vi "AddNewBins.vi"(8 "error in (no error)":errorcluster, 11 "Node Ptr":u64 format="%.0x") -> (0 "error out":errorcluster)   [LabVIEW 2012, in "Histogram Custom Device.lvlib"]
uses:
  Histogram Custom Device.lvlib
  <vilib>/NI Veristand/Custom Device API/Custom Device API.lvlib
  <vilib>/NI Veristand/Custom Device API/Custom Device Channel Type.ctl
  <vilib>/NI Veristand/Custom Device API/Custom Device Channel.ctl
  BinBounds.ctl
  <vilib>/NI Veristand/Custom Device API/Set Item Property (Variant).vi
panel:
  in  "Tag":string
  # "We cant add bins individually,\nwe have to delete all of the existing \nbins and then create new ones"
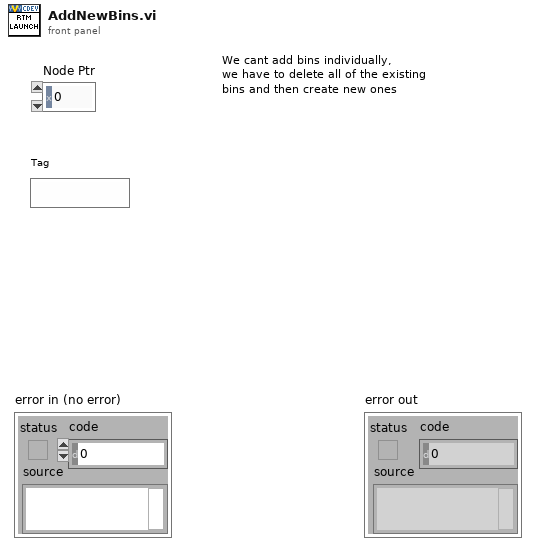
[diagram p1: front panel]
types:
  T1 = typedef "Custom Device API.lvlib/Custom Device Channel.ctl" = cluster{"Type":T2, "Units":string, "Default Value":dbl, "Faultable":bool, "Scalable":bool}
  T2 = typedef "Custom Device API.lvlib/Custom Device Channel Type.ctl" = enum16{"Input", "Output"}
  T3 = typedef "Histogram Custom Device.lvlib/BinBounds.ctl" = cluster{"Bin Counts":i32[], "Upper Bounds":dbl[], "Lower Bounds":dbl[]}
  T4 = typedef "Custom Device API.lvlib/Custom Device Item Ref.ctl" = u64
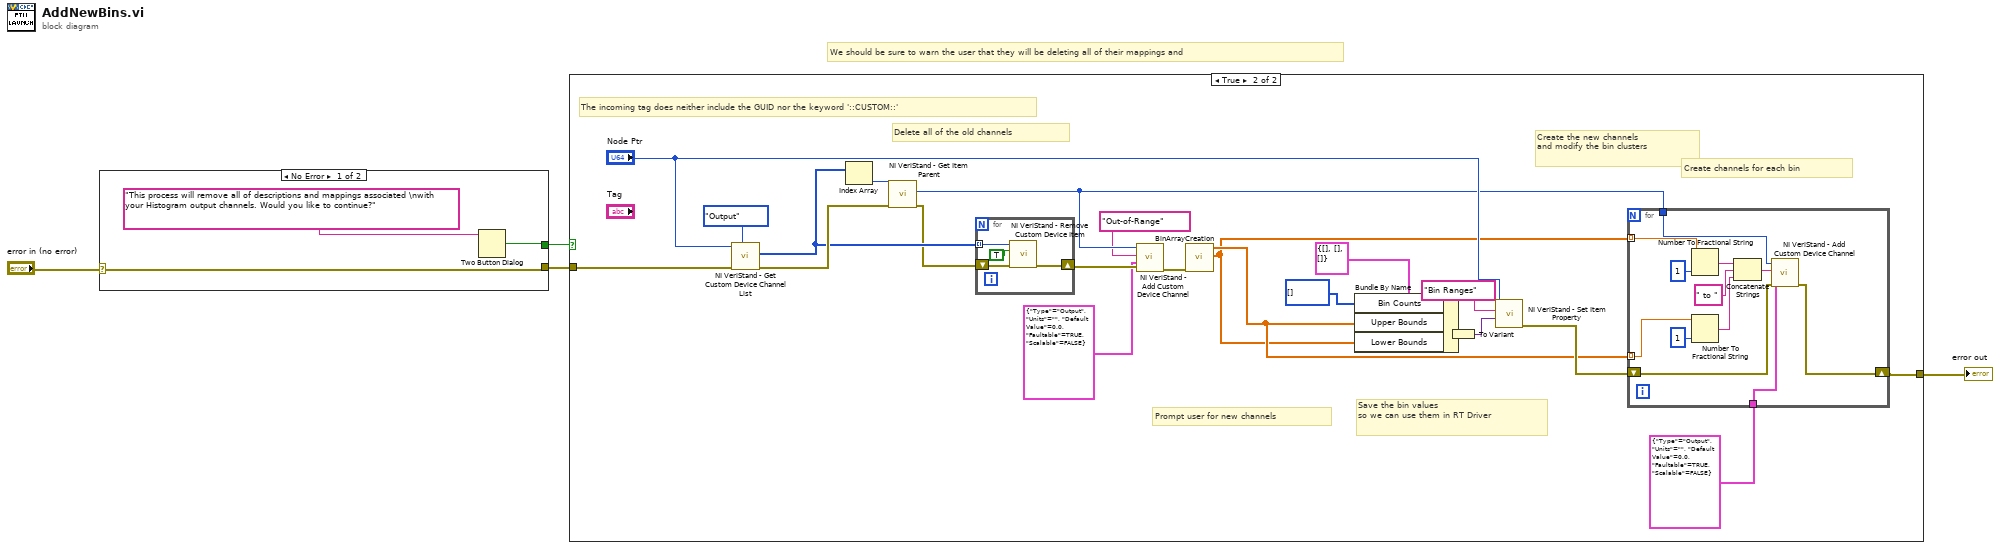
[diagram p0: block diagram]
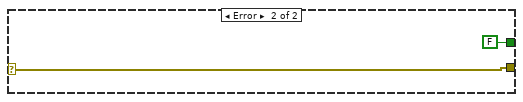
[diagram p3: hidden frame]
diagram:
  # "We should be sure to warn the user that they will be deleting all of their mappings and"
  n1 = case shown="No Error" "error in (no error)" {
    selector: "error in (no error)" -> [w7 w9]
    tunnel: [w7 w9] -> w2
    tunnel: [w5 FALSE ("T button?")] -> w1
    frame No Error {
      n2 = Two Button Dialog(message="This process will remove all of descriptions and mappings associated \nwith your Histogram output channels. Would you like to continue?") -> (T button?=w5:bool)  [unwired: 2 in]
    }
    frame Error {
    }
  }
  n3 = case shown="True" w1 {
    tunnel: [w10 w22] -> w4
    tunnel: w2 -> [w10 w14]
    frame False {
      # "Do nothing"
    }
    frame True {
      # "Create channels for each bin"
      # "Save the bin values\nso we can use them in RT Driver"
      # "Create the new channels\nand modify the bin clusters"
      # "Prompt user for new channels"
      # "Delete all of the old channels"
      # "The incoming tag does neither include the GUID nor the keyword '::CUSTOM::'"
      n4 = call <vilib>:"NI VeriStand - Get Custom Device Channel List.vi"("Channel Type"=Custom_Device_Channel_Type."Output", "error in (no error)"=w14, "Device Ref in"="Node Ptr") -> ("error out"=w21:errorcluster, "Specified Channel Ref List"=w19:T4[])  [unwired: 7 out]
      n5 = Index Array(array=w19) -> (element=w20:T4)  [unwired: 1 in]
      n6 = call <vilib>:"NI VeriStand - Get Item Parent.vi"("error in (no error)"=w21, "Item Ref in"=w20) -> ("error out"=w18:errorcluster, "Parent Ref"=w17:T4)  [unwired: 6 in, 2 out]
      n7 = for {
        tunnel: w19 -> [w47] mode=indexing
        shift-right: [w46] -> w23
        shift-left: w18 -> [w48]
        n8 = call <vilib>:"NI VeriStand - Remove Custom Device Item.vi"("error in (no error)"=w48, "Force Delete (F)"=TRUE, "Item Ref in"=w47) -> ("error out"=w46:errorcluster)  [unwired: 7 in, 1 out]
      }
      n9 = call <vilib>:"NI VeriStand - Add Custom Device Channel.vi"("error in (no error)"=w23, "Channel"=T1 {"Type"=enum."Output", "Units"="", "Default Value"=0.0, "Faultable"=TRUE, "Scalable"=FALSE}, "Channel Name"="Out-of-Range", "Parent Ref in"=w17) -> ("error out"=w13:errorcluster)  [unwired: 4 in, 3 out]
      n10 = call "BinArrayCreation.vi"("error in (no error)"=w13) -> ("Lower Bounds"=w11:dbl[], "Upper Bounds"=w12:dbl[])  [unwired: 8 in, 1 out]
      n11 = Bundle By Name(cluster=T3 {"Bin Counts"=[], "Upper Bounds"=[], "Lower Bounds"=[]} ("Cluster"), "Bin Counts"=i32[] [], "Upper Bounds"=w12, "Lower Bounds"=w11) -> (w26:T3)
      n12 = To Variant(anything=w26) -> (Variant=w27:variant)
      n13 = call-poly <vilib>:"NI VeriStand - Set Item Property.vi"("Value"=w27, "Property Name"="Bin Ranges", "Item Ref in"="Node Ptr") -> ("error out"=w29:errorcluster)  [unwired: 6 in, 2 out]
      n14 = for {
        tunnel: w12 -> [w42] mode=indexing
        tunnel: T1 {"Type"=enum."Output", "Units"="", "Default Value"=0.0, "Faultable"=TRUE, "Scalable"=FALSE} ("Channel") -> [w44]
        shift-right: [w37] -> w22
        shift-left: w29 -> [w43]
        tunnel: w17 -> [w34]
        tunnel: w11 -> [w33] mode=indexing
        n15 = Number To Fractional String(number=w33, precision (6)=i16 1) -> (F-format string=w41:string)  [unwired: 2 in]
        n16 = Number To Fractional String(number=w42, precision (6)=i16 1) -> (F-format string=w40:string)  [unwired: 2 in]
        n17 = Concatenate Strings(w41, " to " ("string"), w40) -> (w38:string)
        n18 = call <vilib>:"NI VeriStand - Add Custom Device Channel.vi"("error in (no error)"=w43, "Channel"=w44, "Channel Name"=w38, "Parent Ref in"=w34) -> ("error out"=w37:errorcluster)  [unwired: 4 in, 3 out]
      }
    }
  }
  "error out" <- w4
